vi "ULx Read (Analog 1D Wfm NChan NSamp).vi"(0 "task in":refnum<k24>, 7 "number of samples per channel":i32=-1, 9 "timeout":dbl=10.0 format="%_4g", 11 "error in":errorcluster) -> (4 "task out":refnum<k24>, 6 "data":waveform(dbl)[](array[waveform]), 15 "error out":errorcluster)   [LabVIEW 2020]
doc: "Reads one or more waveforms from a task that contains one or more analog input channels."
uses:
  C:/Users/William/Documents/LV 2020 builds/LeaktestDAQ/Source-v33/ULx_LV.dll
  ULx_LV.dll
panel:
  # "channel"
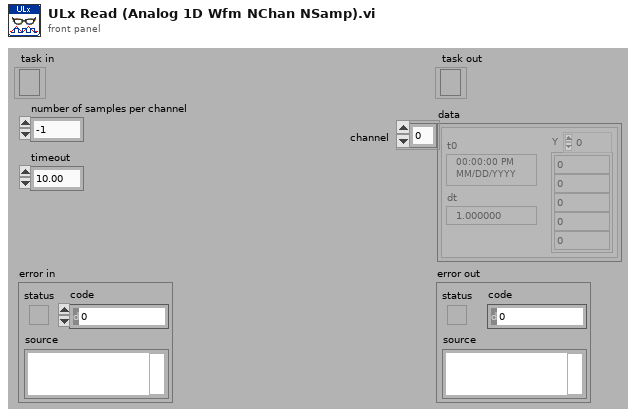
[diagram p1: front panel]
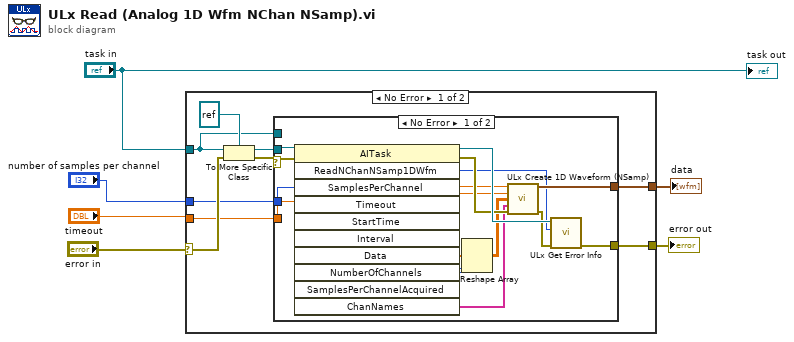
[diagram p0: block diagram]
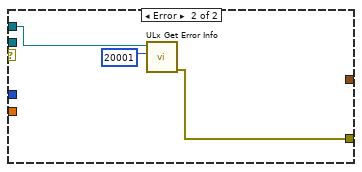
[diagram p2: hidden frame]
diagram:
  n1 = case shown="No Error" "error in" {
    selector: "error in" -> [w15 w36]
    tunnel: "task in" -> [w7 _]
    tunnel: "timeout" -> [w11 _]
    tunnel: [w10 w36] -> w4
    tunnel: "number of samples per channel" -> [w9 _]
    tunnel: [w8 _] -> w1
    frame No Error {
      n2 = To More Specific Class(target class=refnum<k24> refnum, reference=w7, error in=w15) -> (specific class reference=w12:refnum<k24>, error out=w13:errorcluster)
      n3 = case shown="No Error" w13 {
        selector: w13 -> [w31 _]
        tunnel: w12 -> [w32 _]
        tunnel: w11 -> [w29 _]
        tunnel: [w25 w34] -> w10
        tunnel: w9 -> [w28 _]
        tunnel: [w24 _] -> w8
        tunnel: w7 -> [_ w35]
        frame No Error {
          n4 = invoke class="AITask" method="ReadNChanNSamp1DWfm"(reference=w32, error in=w31, "SamplesPerChannel"=w28, "Timeout"=w29) -> (reference out=w30:refnum<k24>, error out=w27:errorcluster, "ReadNChanNSamp1DWfm"=w21:i32, "StartTime"=w23:dbl, "Interval"=w22:dbl, "Data"=w19:dbl[], "NumberOfChannels"=w18:i32, "SamplesPerChannelAcquired"=w20:i32, "ChanNames"=w16:string[])  [unwired: 7 in, 2 out]
          n5 = Reshape Array(w19, w18, w20) -> (w17:dbl[][])
          n6 = call "ULx Create 1D Waveform (NSamp).vi"("t0"=w23, "dt"=w22, "data Array"=w17, "channelName Array"=w16, "error in"=w27) -> ("data"=w24:waveform(dbl)[], "error out"=w26:errorcluster)  [unwired: 9 in]
          n7 = call "ULx Get Error Info.vi"("error in"=w26, "ErrorCode"=w21, "task in"=w30) -> ("error out"=w25:errorcluster)  [unwired: 8 in]
        }
        frame Error {
          n8 = call "ULx Get Error Info.vi"("ErrorCode"=20001, "task in"=w35) -> ("error out"=w34:errorcluster)  [unwired: 9 in]
        }
      }
    }
    frame Error {
    }
  }
  "error out" <- w4
  "data" <- w1
  "task out" <- "task in"
